vi "Compl Notif with Error Msg.vi"() -> ()   [LabVIEW 2023, in "Async Methods Actor.lvlib"]
uses:
  Async Methods Actor.lvlib
  Async Methods Actor Messages/Compl Notif with Error Msg/Compl Notif with Error Msg.lvclass
panel:
  in  "Compl Notif with Error Msg.lvclass":refnum<class "Compl Notif with Error Msg.lvclass">
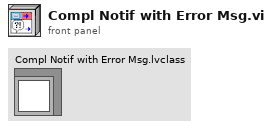
[diagram p1: front panel]
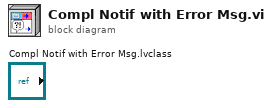
[diagram p0: block diagram]
diagram:
